vi "CreatIO.vi"(8 "error in (no error)":errorcluster, 11 "address":string="USB-4761,BID#0/port0") -> (0 "error out":errorcluster, 2 "IO":i32, 3 "TCP Out":refnum<k5>)   [LabVIEW 2014]
panel:
  in  "TCP In":refnum<k5>
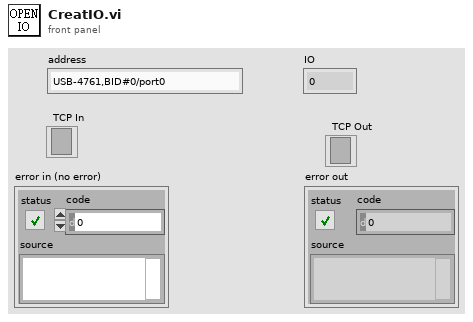
[diagram p1: front panel]
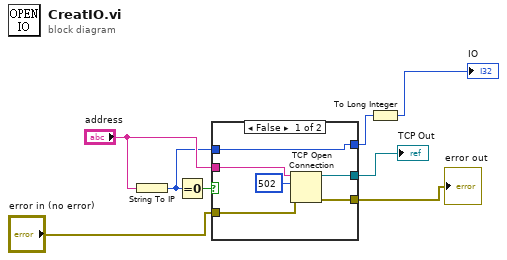
[diagram p0: block diagram]
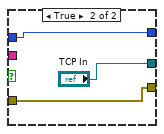
[diagram p2: hidden frame]
diagram:
  n1 = String To IP(1:"address") -> (0:w4:u32)
  n2 = Equal To 0?(x=w4) -> (x = 0?=w6:bool)
  n3 = case shown="False" w6 {
    tunnel: "address" -> [w14 _]
    tunnel: "error in (no error)" -> [w13 w16]
    tunnel: [w11 "TCP In"] -> w1
    tunnel: [w10 w16] -> w7
    tunnel: w4 -> [w9 w15]
    tunnel: [w9 w15] -> w3
    frame False {
      n4 = TCP Open Connection(address=w14, remote port or service name=u16 502, error in (no error)=w13) -> (connection ID=w11:refnum<k5>, error out=w10:errorcluster)  [unwired: 2 in]
    }
    frame True {
    }
  }
  "error out" <- w7
  "TCP Out" <- w1
  n5 = To Long Integer(number=w3) -> (32bit integer=→"IO":i32)
